vi "Main.vi"() -> ()   [LabVIEW 2021]
uses:
  Controls/UI References.ctl
  Controls/App Data.ctl
  <extravilib>/ChannelInstances/Event Messenger-c(str,var)/Instantiate.vi
  <extravilib>/ChannelInstances/Event Messenger-c(str,var)/))Channel.vi
  <extravilib>/ChannelInstances/Event Messenger-c(str,var).lvlib
panel:
  out "Temp 3":dbl
  out "Temp 2":dbl
  out "Temp 1":dbl
  in  "Stop":bool
  in  "Start":bool
  out "Recording?":bool
  in  "Record?":bool
  out "File Path":path
  in  "Confirm":bool
  out "Pressure":dbl
  in  "VISA resource name":refnum<visa-resource-name>
  out "Waveform Chart":dbl(graph)
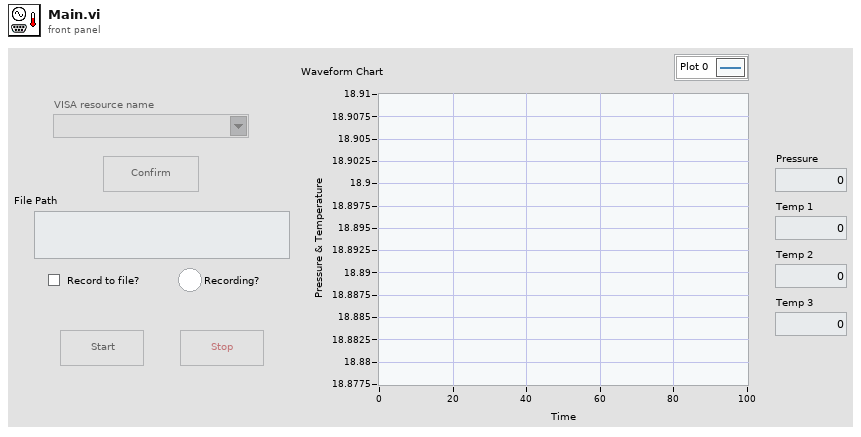
[diagram p1: front panel]
types:
  T1 = typedef "App Data.ctl" = cluster{"VISA resource name":refnum<visa-resource-name>, "File Refnum":refnum<file>}
  T2 = typedef "UI References.ctl" = cluster{"VISA resource name":refnum<vi>, "Confirm":refnum<vi>, "File Path":refnum<vi>, "Record?":refnum<vi>, "Recording?":refnum<vi>, "Start":refnum<vi>, "Stop":refnum<vi>, "Waveform Chart":refnum<vi>, "Pressure":refnum<vi>, "Temp 1":refnum<vi>, "Temp 2":refnum<vi>, "Temp 3":refnum<vi>}
  T3 = typedef "Event Messenger-c(str,var).lvlib/))Channel.ctl" = refnum<queue>
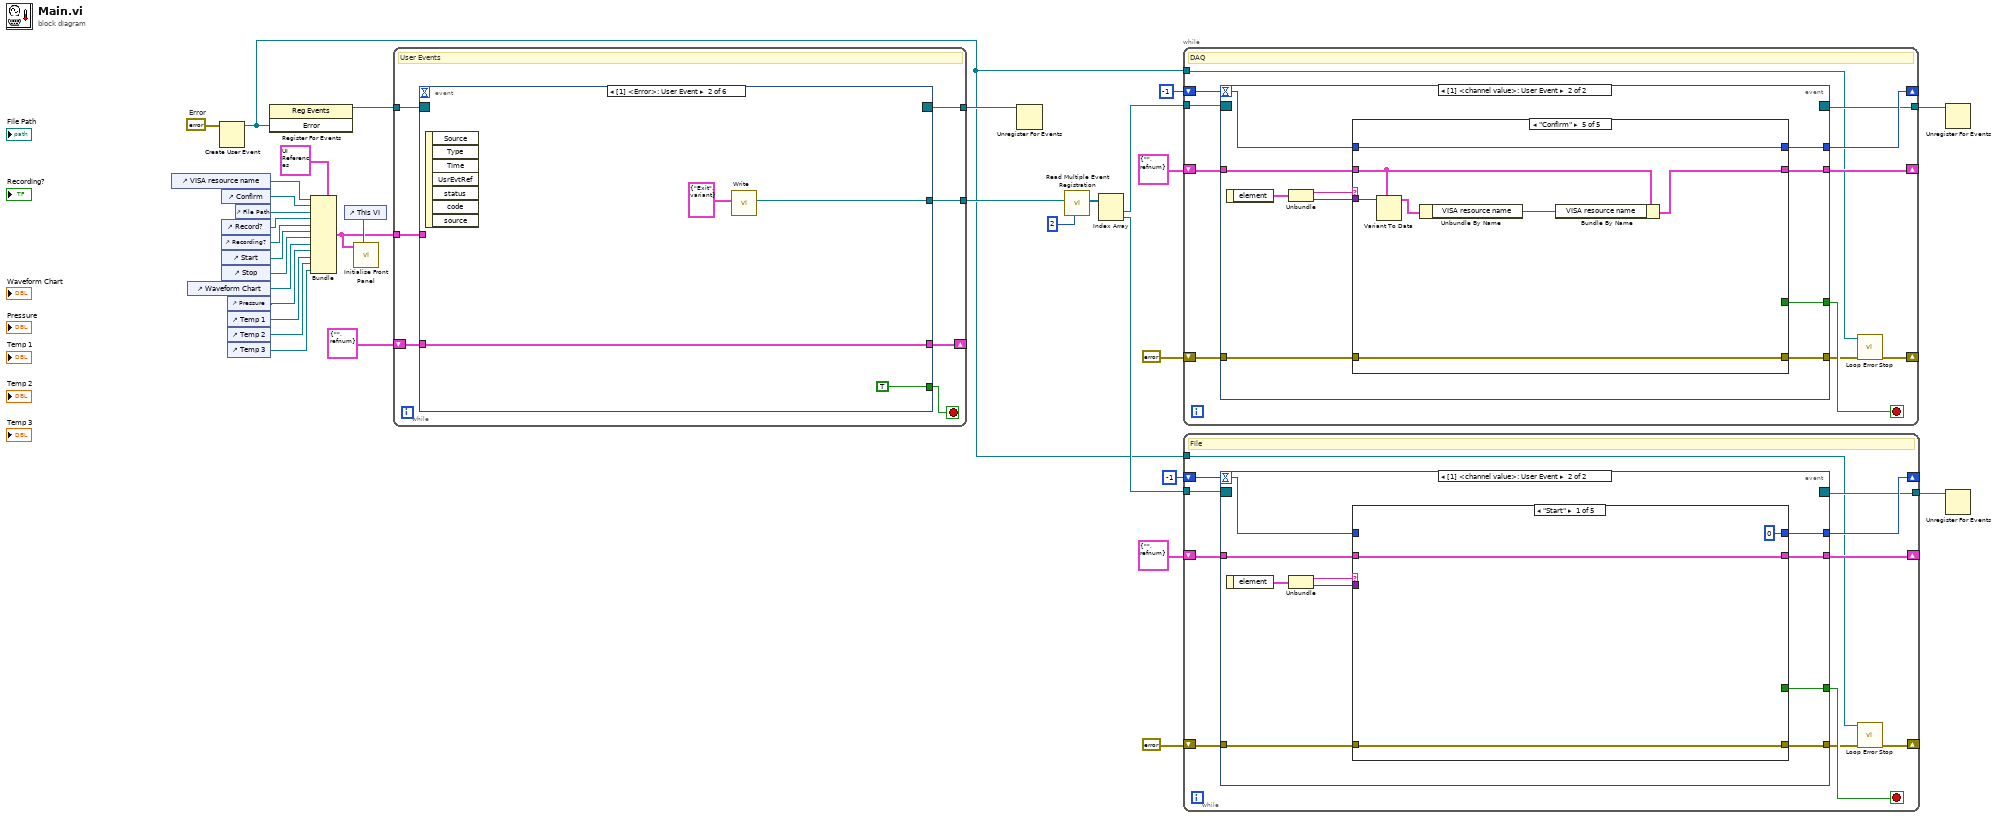
[diagram p0: block diagram]
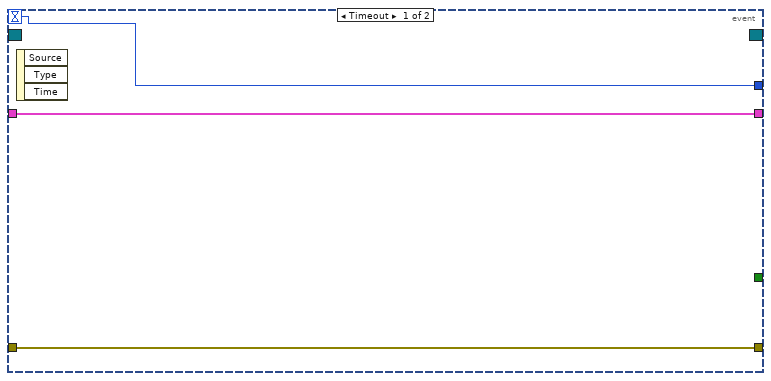
[diagram p2: hidden frame]
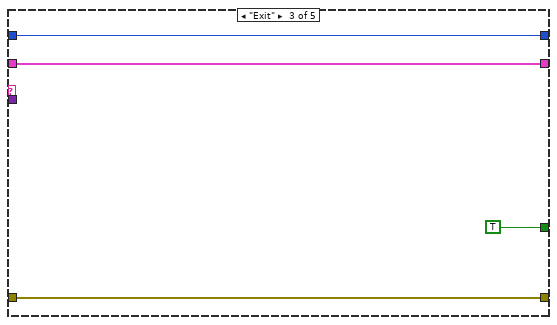
[diagram p4: hidden frame]
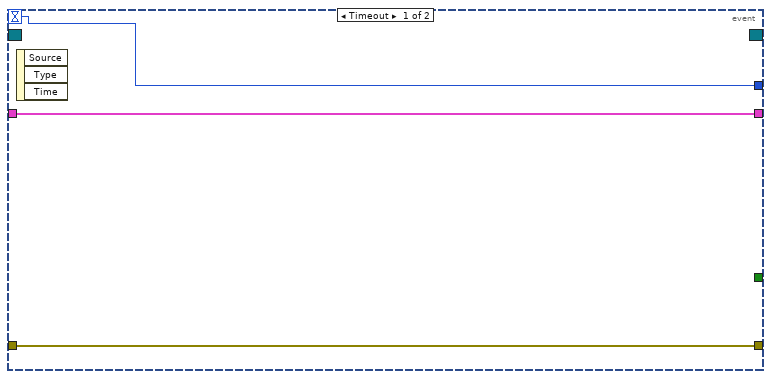
[diagram p7: hidden frame]
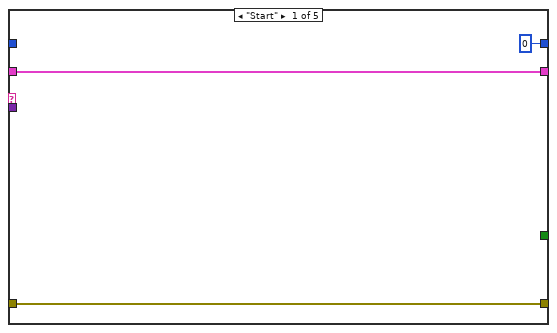
[diagram p8: hidden frame]
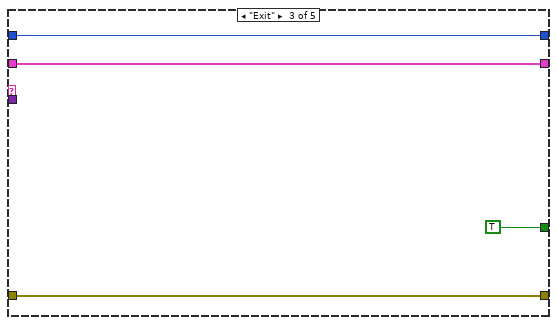
[diagram p10: hidden frame]
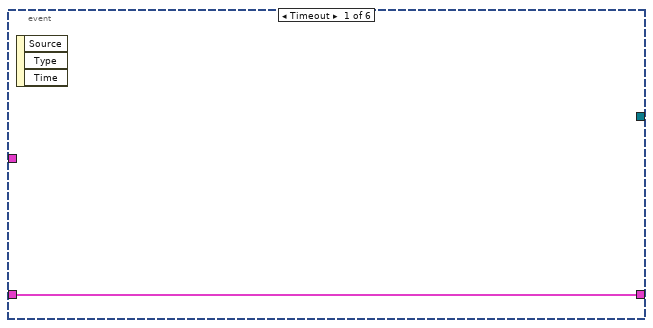
[diagram p12: hidden frame]
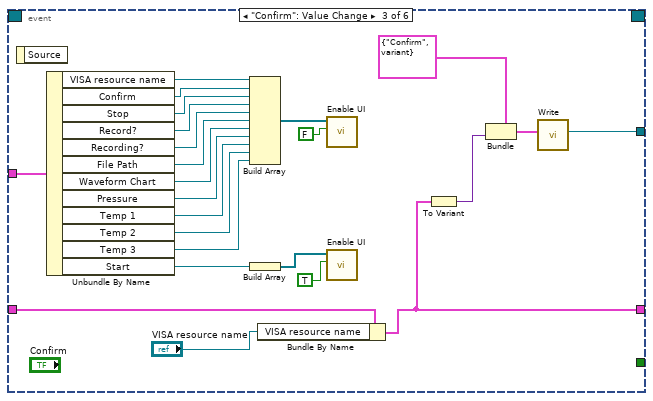
[diagram p13: hidden frame]
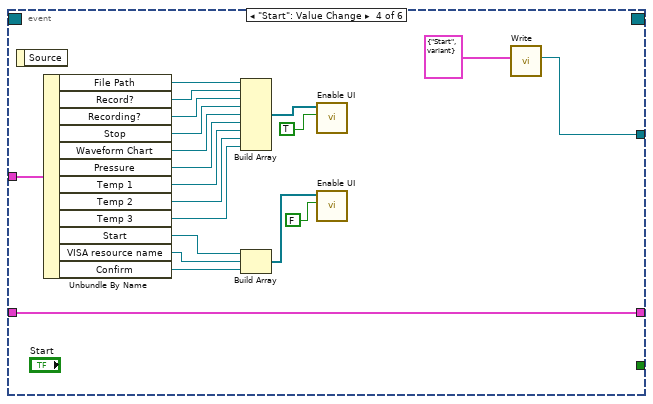
[diagram p14: hidden frame]
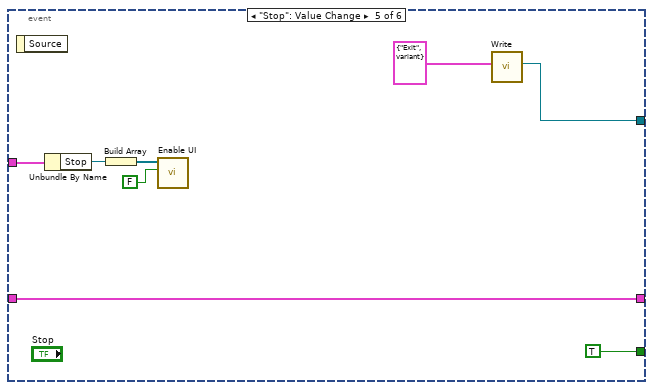
[diagram p15: hidden frame]
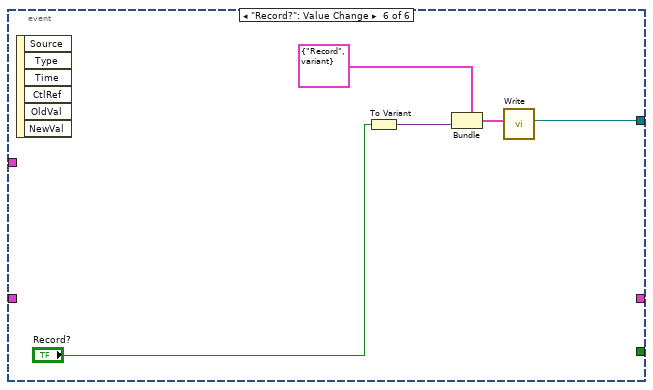
[diagram p16: hidden frame]
diagram:
  w6 = errorcluster {"status"=FALSE, "code"=0, "source"=""}  # Error
  n1 = control-ref of="VISA resource name"() -> (w33:refnum<vi>)
  n2 = control-ref of="Waveform Chart"() -> (w26:refnum<vi>)
  n3 = Create User Event(user event datatype=w6) -> (user event=w3:refnum<user-event>)  [unwired: 1 in, 1 out]
  n4 = control-ref of="Confirm"() -> (w32:refnum<vi>)
  n5 = control-ref of="Record?"() -> (w30:refnum<vi>)
  n6 = control-ref of="Recording?"() -> (w29:refnum<vi>)
  n7 = control-ref of="Start"() -> (w28:refnum<vi>)
  n8 = control-ref of="Stop"() -> (w27:refnum<vi>)
  n9 = control-ref of="Pressure"() -> (w25:refnum<vi>)
  n10 = control-ref of="Temp 1"() -> (w24:refnum<vi>)
  n11 = control-ref of="Temp 2"() -> (w23:refnum<vi>)
  n12 = control-ref of="Temp 3"() -> (w22:refnum<vi>)
  n13 = control-ref of="File Path"() -> (w31:refnum<vi>)
  n14 = register-events(w3) -> (reference out=w5:refnum<event-registration>)  [unwired: 2 in, 1 out]
  n15 = Bundle(cluster=T2 {"VISA resource name"=refnum, "Confirm"=refnum, "File Path"=refnum, "Record?"=refnum, "Recording?"=refnum, "Start"=refnum, "Stop"=refnum, "Waveform Chart"=refnum, "Pressure"=refnum, "Temp 1"=refnum, "Temp 2"=refnum, "Temp 3"=refnum} ("UI Ref"), "VISA resource name"=w33, "Confirm"=w32, "File Path"=w31, "Record?"=w30, "Recording?"=w29, "Start"=w28, "Stop"=w27, "Waveform Chart"=w26, "Pressure"=w25, "Temp 1"=w24, "Temp 2"=w23, "Temp 3"=w22) -> (w19:T2)
  n16 = control-ref of="This VI"() -> (w20:refnum<vi>)
  n17 = call "Initialise Front Panel.vi"("This VI"=w20, "UI Ref"=w19) -> ()  [unwired: 9 in, 1 out]
  n18 = while {
    tunnel: w19 -> [w40]
    shift-right: [w37] -> _
    shift-left: T1 {"VISA resource name"="", "File Refnum"=refnum} ("App Data") -> [w38]
    tunnel: [w36] -> w17
    tunnel: w5 -> [w35]
    tunnel: [w34] -> w4
    stop <- w39 stop-if-true
    # "User Events"
    n19 = event shown="[1] <Error>: User Event" {
      selector: w35 -> [_ _ _ _ _ _]
      dyn-events: [_ _ _ _ _ _] -> w34
      timeout: _ -> [_ _ _ _ _ _]
      tunnel: w40 -> [_ _ w69 w89 w96 _]
      tunnel: [_ TRUE _ _ TRUE _] -> w39
      tunnel: w38 -> [w41 w43 w52 w72 w92 _]
      tunnel: [w41 w43 w50 w72 w92 _] -> w37
      tunnel: [_ w44 w46 w70 w90 w98] -> w36
      event Timeout {
        n20 = event-data() -> ()  [unwired: 1 in, 3 out]
      }
      event User Event {
        n21 = event-data() -> ()  [unwired: 1 in, 7 out]
        n22 = call <extravilib>:"Write.vi"("element"=cluster{string, variant} {"Exit", variant}) -> ("channel"=w44:T3)  [unwired: 9 in, 1 out]
      }
      event "Confirm": Value Change {
        n23 = event-data() -> ()  [unwired: 1 in, 1 out]
        n24 = Unbundle By Name(w69) -> ("VISA resource name"=w68:refnum<vi>, "Confirm"=w67:refnum<vi>, "Stop"=w66:refnum<vi>, "Record?"=w65:refnum<vi>, "Recording?"=w64:refnum<vi>, "File Path"=w63:refnum<vi>, "Waveform Chart"=w62:refnum<vi>, "Pressure"=w61:refnum<vi>, "Temp 1"=w60:refnum<vi>, "Temp 2"=w59:refnum<vi>, "Temp 3"=w58:refnum<vi>, "Start"=w57:refnum<vi>)
        n25 = Build Array(w68, w67, w66, w65, w64, w63, w62, w61, w60, w59, w58) -> (w56:refnum<vi>[])
        n26 = Build Array(w57) -> (w55:refnum<vi>[])
        n27 = Bundle By Name(cluster=w52, "VISA resource name"="VISA resource name") -> (w50:T1)
        n28 = call "Enable UI.vi"("Enable?"=FALSE, "output cluster"=w56) -> ()  [unwired: 9 in, 1 out]
        n29 = call "Enable UI.vi"("Enable?"=TRUE, "output cluster"=w55) -> ()  [unwired: 9 in, 1 out]
        n30 = To Variant(anything=w50) -> (Variant=w48:variant)
        n31 = Bundle(cluster=cluster{string, variant} {"Confirm", variant}, w48) -> (w47:cluster{string, variant})  [unwired: 1 in]
        n32 = call <extravilib>:"Write.vi"("element"=w47) -> ("channel"=w46:T3)  [unwired: 9 in, 1 out]
      }
      event "Start": Value Change {
        n33 = event-data() -> ()  [unwired: 1 in, 1 out]
        n34 = Unbundle By Name(w89) -> ("File Path"=w88:refnum<vi>, "Record?"=w87:refnum<vi>, "Recording?"=w86:refnum<vi>, "Stop"=w85:refnum<vi>, "Waveform Chart"=w84:refnum<vi>, "Pressure"=w83:refnum<vi>, "Temp 1"=w82:refnum<vi>, "Temp 2"=w81:refnum<vi>, "Temp 3"=w80:refnum<vi>, "Start"=w79:refnum<vi>, "VISA resource name"=w74:refnum<vi>, "Confirm"=w73:refnum<vi>)
        n35 = Build Array(w88, w87, w86, w85, w84, w83, w82, w81, w80) -> (w78:refnum<vi>[])
        n36 = Build Array(w79, w74, w73) -> (w77:refnum<vi>[])
        n37 = call "Enable UI.vi"("Enable?"=TRUE, "output cluster"=w78) -> ()  [unwired: 9 in, 1 out]
        n38 = call "Enable UI.vi"("Enable?"=FALSE, "output cluster"=w77) -> ()  [unwired: 9 in, 1 out]
        n39 = call <extravilib>:"Write.vi"("element"=cluster{string, variant} {"Start", variant}) -> ("channel"=w70:T3)  [unwired: 9 in, 1 out]
      }
      event "Stop": Value Change {
        n40 = event-data() -> ()  [unwired: 1 in, 1 out]
        n41 = Unbundle By Name(w96) -> ("Stop"=w95:refnum<vi>)
        n42 = Build Array(w95) -> (w94:refnum<vi>[])
        n43 = call "Enable UI.vi"("Enable?"=FALSE, "output cluster"=w94) -> ()  [unwired: 9 in, 1 out]
        n44 = call <extravilib>:"Write.vi"("element"=cluster{string, variant} {"Exit", variant}) -> ("channel"=w90:T3)  [unwired: 9 in, 1 out]
      }
      event "Record?": Value Change {
        n45 = event-data() -> ()  [unwired: 1 in, 6 out]
        n46 = To Variant(anything="Record?") -> (Variant=w100:variant)
        n47 = Bundle(cluster=cluster{string, variant} {"Record", variant}, w100) -> (w99:cluster{string, variant})  [unwired: 1 in]
        n48 = call <extravilib>:"Write.vi"("element"=w99) -> ("channel"=w98:T3)  [unwired: 9 in, 1 out]
      }
    }
  }
  n49 = Unregister For Events(event registration refnum=w4) -> ()  [unwired: 1 in, 1 out]
  n50 = call <extravilib>:"Read Multiple Event Registration.vi"("number of event structures"=u16 2, "channel"=w17) -> ("event registration refnums"=w15:refnum<event-registration>[])  [unwired: 9 in]
  n51 = Index Array(array=w15) -> (element #1=w14:refnum<event-registration>, element #2=w8:refnum<event-registration>)  [unwired: 2 in]
  n52 = while {
    tunnel: w14 -> [w113]
    shift-right: [w111] -> _
    shift-left: T1 {"VISA resource name"="", "File Refnum"=refnum} ("App Data") -> [w112]
    shift-right: [w108] -> _
    shift-left: -1 -> [w109]
    tunnel: [w107] -> w11
    tunnel: w3 -> [w103]
    shift-right: [w104] -> _
    shift-left: errorcluster {"status"=FALSE, "code"=0, "source"=""} ("Error") -> [w106]
    stop <- w110 stop-if-true
    # "DAQ"
    n53 = event shown="[1] <channel value>: User Event" {
      selector: w113 -> [_ _]
      dyn-events: [_ _] -> w107
      timeout: w109 -> [w115 w120]
      tunnel: w112 -> [w116 w123]
      tunnel: [w116 w122] -> w111
      tunnel: [_ w121] -> w110
      tunnel: [w115 w119] -> w108
      tunnel: w106 -> [w114 w118]
      tunnel: [w114 w117] -> w105
      event Timeout {
        n54 = event-data() -> ()  [unwired: 1 in, 3 out]
      }
      event User Event {
        n55 = event-data() -> ("element"=w126:cluster{string, "Data":variant})  [unwired: 1 in]
        n56 = Unbundle(w126) -> (w125:string, "Data"=w124:variant)
        n57 = case shown="\"Confirm\"" w125 {
          tunnel: w124 -> [_ _ _ _ w144]
          tunnel: w123 -> [w129 w132 w136 w139 w142]
          tunnel: [w129 w132 w136 w139 w140] -> w122
          tunnel: [_ _ TRUE _ _] -> w121
          tunnel: w120 -> [_ w131 w134 w138 w146]
          tunnel: [0 w131 w134 w138 w146] -> w119
          tunnel: w118 -> [w127 w130 w133 w137 w145]
          tunnel: [w127 w130 w133 w137 w145] -> w117
          frame "Start" {
          }
          frame "Record" {
          }
          frame "Exit" {
          }
          frame Default {
          }
          frame "Confirm" {
            n58 = Variant To Data(type=w142, Variant=w144) -> (data=w143:T1)  [unwired: 1 in, 1 out]
            n59 = Unbundle By Name(w143) -> ("VISA resource name"=w141:refnum<visa-resource-name>)
            n60 = Bundle By Name(cluster=w142, "VISA resource name"=w141) -> (w140:T1)
          }
        }
      }
    }
    n61 = call "Loop Error Stop.vi"("error in"=w105, "user event"=w103) -> ("error out"=w104:errorcluster)  [unwired: 9 in]
  }
  n62 = while {
    tunnel: w8 -> [w157]
    shift-right: [w155] -> _
    shift-left: T1 {"VISA resource name"="", "File Refnum"=refnum} ("App Data") -> [w156]
    shift-right: [w152] -> _
    shift-left: -1 -> [w153]
    tunnel: [w151] -> w10
    tunnel: w3 -> [w147]
    shift-right: [w148] -> _
    shift-left: errorcluster {"status"=FALSE, "code"=0, "source"=""} ("Error") -> [w150]
    stop <- w154 stop-if-true
    # "File"
    n63 = event shown="[1] <channel value>: User Event" {
      selector: w157 -> [_ _]
      dyn-events: [_ _] -> w151
      timeout: w153 -> [w159 w164]
      tunnel: w156 -> [w160 w167]
      tunnel: [w160 w166] -> w155
      tunnel: [_ w165] -> w154
      tunnel: [w159 w163] -> w152
      tunnel: w150 -> [w158 w161]
      tunnel: [w158 w162] -> w149
      event Timeout {
        n64 = event-data() -> ()  [unwired: 1 in, 3 out]
      }
      event User Event {
        n65 = event-data() -> ("element"=w170:cluster{string, "Data":variant})  [unwired: 1 in]
        n66 = Unbundle(w170) -> (w169:string, "Data"=w168:variant)
        n67 = case shown="\"Start\"" w169 {
          tunnel: w168 -> [_ _ _ _ _]
          tunnel: w167 -> [w173 w176 w180 w183 w186]
          tunnel: [w173 w176 w180 w183 w186] -> w166
          tunnel: [_ _ TRUE _ _] -> w165
          tunnel: w164 -> [_ w175 w178 w182 w185]
          tunnel: [0 w175 w178 w182 w185] -> w163
          tunnel: [w171 w174 w177 w181 w184] -> w162
          tunnel: w161 -> [w171 w174 w177 w181 w184]
          frame "Start" {
          }
          frame "Record" {
          }
          frame "Exit" {
          }
          frame Default {
          }
          frame "Confirm" {
          }
        }
      }
    }
    n68 = call "Loop Error Stop.vi"("error in"=w149, "user event"=w147) -> ("error out"=w148:errorcluster)  [unwired: 9 in]
  }
  n69 = Unregister For Events(event registration refnum=w11) -> ()  [unwired: 1 in, 1 out]
  n70 = Unregister For Events(event registration refnum=w10) -> ()  [unwired: 1 in, 1 out]
